vi "CALC_TRAN_TIME_STAT_ON_OFF.vi"(0 "VISA IN":refnum<visa-resource-name>, 1 "Time Domain ON/OFF":bool, 5 "error in":errorcluster, 7 "Channel":i32) -> (14 "VISA Out":refnum<visa-resource-name>, 19 "error out":errorcluster)   [LabVIEW 2018, in "PNA-X.lvlib"]
doc: "CALCulate<cnum>:TRANsform:TIME:STATe <ON | OFF> \n(Read-Write) Turns the time domain transform capability ON or OFF. \nSee Critical Note \nNote: Sweep type must be set to Linear Frequency in order to use Time Domain Transform. \nParameters \n<cnum> Channel number of the measurement. There must be a selected measurement \non that channel. If unspecified, <cnum> is set to 1. \n<ON|OFF> ON (or 1) - turns time domain ON. \nOFF (or 0) - turns time domain OFF. \nExamples CALC:TRAN:TIME:STAT ON \ncalculate2:transform:time:state off \nQuery Syntax CALCulate<cnum>:TRANsform:TIME:STATe? \nReturn Type Boolean (1 = ON, 0 = OFF) \nDefault OFF"
uses:
  PNA-X.lvlib
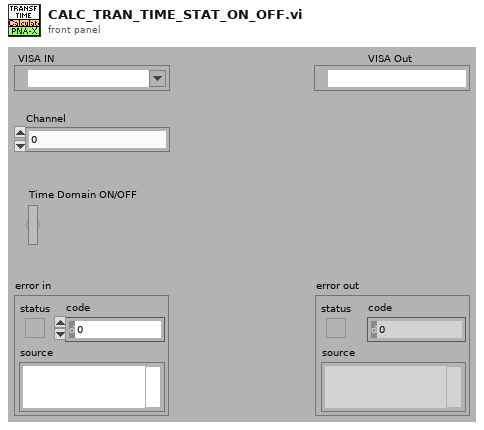
[diagram p1: front panel]
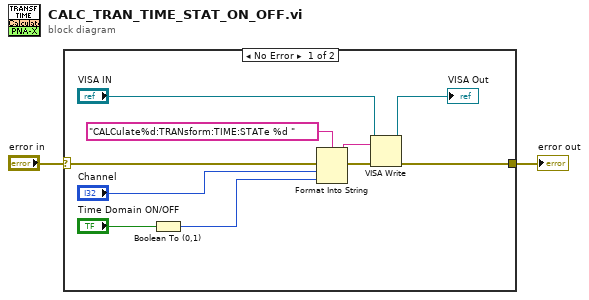
[diagram p0: block diagram]
diagram:
  n1 = case shown="No Error" "error in" {
    selector: "error in" -> [w12 w13]
    tunnel: [w7 w13] -> w1
    frame No Error {
      n2 = Boolean To (0,1)(Boolean="Time Domain ON/OFF") -> (0, 1=w3:i16)
      n3 = Format Into String(format string="CALCulate%d:TRANsform:TIME:STATe %d " ("Cmdline"), error in=w12, "Channel", w3) -> (resulting string=w10:string, error out=w11:errorcluster)  [unwired: 1 in]
      n4 = VISA Write(VISA resource name="VISA IN", write buffer=w10, error in (no error)=w11) -> (VISA resource name out=→"VISA Out":refnum<visa-resource-name>, error out=w7:errorcluster)  [unwired: 1 out]
    }
    frame Error {
    }
  }
  "error out" <- w1
